vi "TalonLights.vi"(8 "error in":errorcluster, 11 "LED Lights Ref In":T1={"I2CDevRef"={"DevStatus"={"status"=FALSE, "code"=0, "source"=""}, "Device Address"=0, "Handle"=0, "I2C Bus"=enum."Invalid"}} {"I2CDevRef"."Device Address" format="%.0x"}) -> (0 "error out":errorcluster, 3 "LED Lights Ref Out":T1={"I2CDevRef"={"DevStatus"={"status"=FALSE, "code"=0, "source"=""}, "Device Address"=0, "Handle"=0, "I2C Bus"=enum."Invalid"}} {"I2CDevRef"."Device Address" format="%.0x"})   [LabVIEW 2015]
uses:
  LED Lights Ref.ctl
  <vilib>/Rock Robotics/WPI/I2C/WPI_I2CDevRef.ctl
  <vilib>/Rock Robotics/SystemInterfaces/i2clib/i2c_bus.ctl
  Drive/Implementation/RobotDriveGlobal.vi
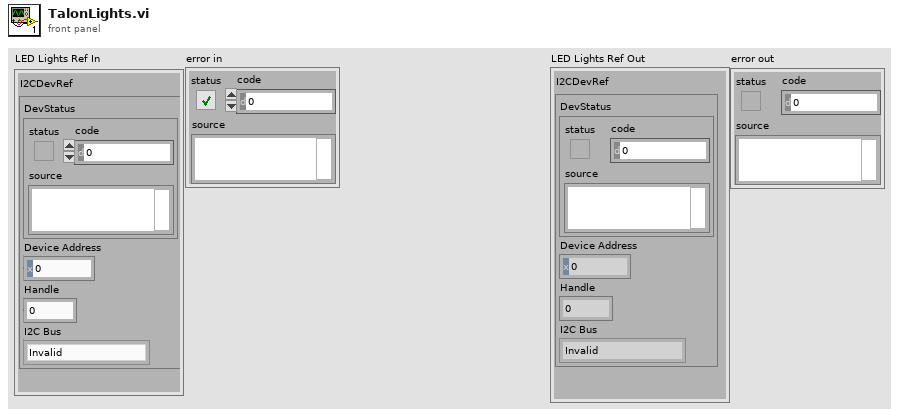
[diagram p1: front panel]
types:
  T1 = typedef "LED Lights Ref.ctl" = cluster{"I2CDevRef":T2}
  T2 = typedef "WPI_I2CDevRef.ctl" = cluster{"DevStatus":errorcluster, "Device Address":u8, "Handle":i32, "I2C Bus":T3}
  T3 = typedef "i2c_bus.ctl" = enum16{"I2C On-Board", "I2C MXP", "Invalid"}
  T4 = typedef "Drive Error Type Def.ctl" = cluster{"Front Left":errorcluster, "Front Right":errorcluster, "Rear Left":errorcluster, "Rear Right":errorcluster}
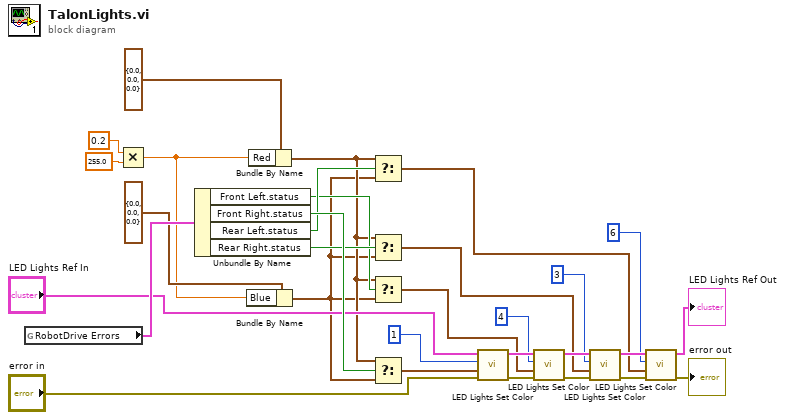
[diagram p0: block diagram]
diagram:
  n1 = global read "RobotDriveGlobal.vi" "RobotDrive Errors"() -> (w30:T4)
  n2 = Multiply(x=0.2, y=255.0 ("Red")) -> (x*y=w2:dbl)
  n3 = Unbundle By Name(w30) -> ("Front Left.status"=w13:bool, "Front Right.status"=w29:bool, "Rear Left.status"=w15:bool, "Rear Right.status"=w14:bool)
  n4 = Bundle By Name(cluster=cluster{"Red":dbl, "Green":dbl, "Blue":dbl} {"Red"=0.0, "Green"=0.0, "Blue"=0.0} ("Color"), "Blue"=w2) -> (w4:cluster{"Red":dbl, "Green":dbl, "Blue":dbl})
  n5 = Bundle By Name(cluster=cluster{"Red":dbl, "Green":dbl, "Blue":dbl} {"Red"=0.0, "Green"=0.0, "Blue"=0.0} ("Color"), "Red"=w2) -> (w11:cluster{"Red":dbl, "Green":dbl, "Blue":dbl})
  n6 = Select(t=w11, s=w15, f=w4) -> (s? t:f=w16:cluster{"Red":dbl, "Green":dbl, "Blue":dbl})
  n7 = Select(t=w11, s=w14, f=w4) -> (s? t:f=w17:cluster{"Red":dbl, "Green":dbl, "Blue":dbl})
  n8 = Select(t=w11, s=w13, f=w4) -> (s? t:f=w18:cluster{"Red":dbl, "Green":dbl, "Blue":dbl})
  n9 = Select(t=w11, s=w29, f=w4) -> (s? t:f=w19:cluster{"Red":dbl, "Green":dbl, "Blue":dbl})
  n10 = call "LED Lights Set Color.vi"("error in"="error in", "Color"=w19, "Light ID"=1 ("Motor ID"), "LED Lights Ref In"="LED Lights Ref In") -> ("error out"=w9:errorcluster, "LED Lights Ref Out"=w26:T1)  [unwired: 6 in]
  n11 = call "LED Lights Set Color.vi"("error in"=w9, "Color"=w18, "Light ID"=4 ("Motor ID"), "LED Lights Ref In"=w26) -> ("error out"=w8:errorcluster, "LED Lights Ref Out"=w25:T1)  [unwired: 6 in]
  n12 = call "LED Lights Set Color.vi"("error in"=w8, "Color"=w17, "Light ID"=3 ("Motor ID"), "LED Lights Ref In"=w25) -> ("error out"=w7:errorcluster, "LED Lights Ref Out"=w24:T1)  [unwired: 6 in]
  n13 = call "LED Lights Set Color.vi"("error in"=w7, "Color"=w16, "Light ID"=6 ("Motor ID"), "LED Lights Ref In"=w24) -> ("error out"=→"error out":errorcluster, "LED Lights Ref Out"=→"LED Lights Ref Out":T1)  [unwired: 6 in]
